vi "Abort Mission and RTH.vi"(8 "Error In":errorcluster, 11 "Aircraft Index":u8) -> (0 "Error Out":errorcluster)   [LabVIEW 2014]
uses:
  Aircraft Information/Sub VI/Get Aircraft Waypoints.vi
  Commands/Mission Planning/MISSION_ITEM SubVI/MISSION_ITEM Jump.vi
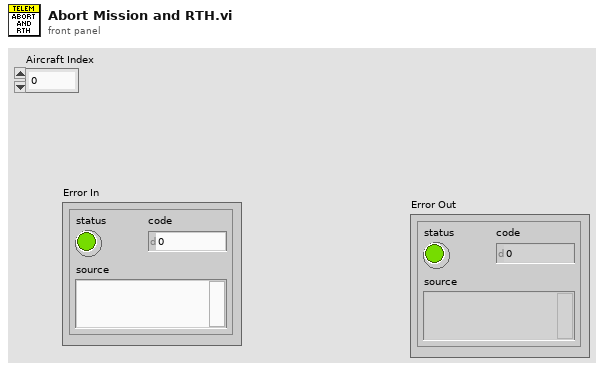
[diagram p1: front panel]
types:
  T1 = typedef "MAVLINK Mav Frame.ctl" = enum8{"GLOBAL", "LOCAL NED", "MISSION", "GLOBAL RELATIVE ALT", "LOCAL ENU", "GLOBAL INT", "GLOBAL RELATIVE ALT INT", "LOCAL OFFSET NED", "BODY NED", "BODY OFFSET NED", "GLOBAL TERRAIN ALT", "GLOBAL TERRAIN ALT INT"}
  T2 = cluster{"target_system":u8, "target_component":u8, "sequence":u16, "frame":T1, "command":u16, "current":bool, "autocontinue":bool, "param1":sgl, "param2":sgl, "param3":sgl, "param4":sgl, "x":sgl, "y":sgl, "z":sgl}[]
  T3 = typedef "MAVLINK Mission Item.ctl" = cluster{"target_system":u8, "target_component":u8, "sequence":u16, "frame":T1, "command":u16, "current":bool, "autocontinue":bool, "param1":sgl, "param2":sgl, "param3":sgl, "param4":sgl, "Lat":sgl, "Lon":sgl, "Altitude (m)":sgl}
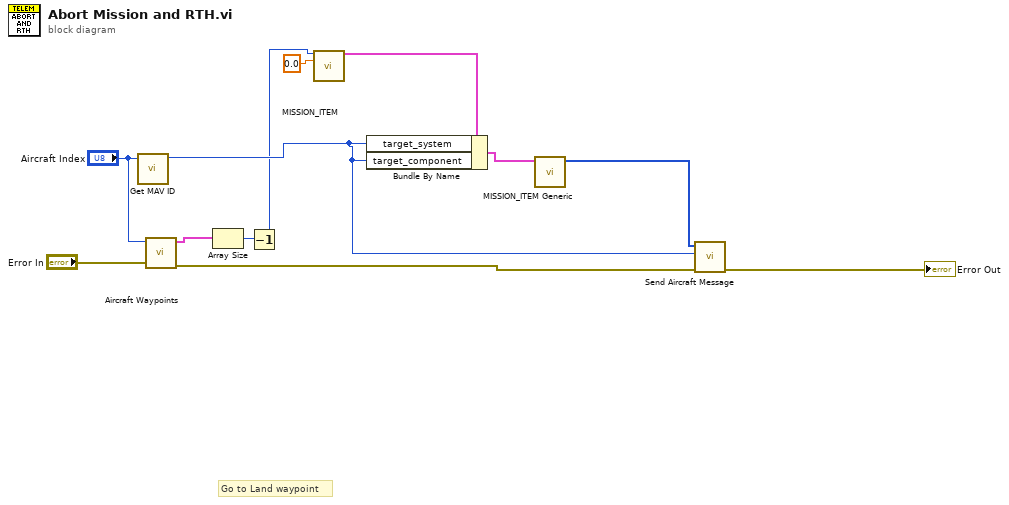
[diagram p0: block diagram]
diagram:
  # "Go to Land waypoint"
  n1 = call "Get MAV ID.vi"("Aircraft Index"="Aircraft Index") -> ("Aircraft ID"=w9:u8)  [unwired: 10 in]
  n2 = call-poly "Aircraft Waypoints.vi"("Error In"="Error In", "Aircraft ID"="Aircraft Index") -> ("Error Out"=w6:errorcluster, "Waypoints Out"=w4:T2)  [unwired: 8 in]
  n3 = Array Size(array=w4) -> (size(s)=w3:i32)
  n4 = Decrement(x=w3) -> (x-1=w2:i32)
  n5 = call-poly "MISSION_ITEM.vi"("Waypoint to jump to"=w2, "Number of times to repeat"=sgl 0.0) -> ("Mission Item"=w12:T3)  [unwired: 13 in]
  n6 = Bundle By Name(cluster=w12, "target_system"=w9, "target_component"=w9) -> (w11:T3)
  n7 = call "MISSION_ITEM Generic.vi"("MISSION_ITEM"=w11) -> ("MAVLink Message"=w10:u8[])  [unwired: 10 in]
  n8 = call "Send Aircraft Message.vi"("error in (no error)"=w6, "Aircraft ID"=w9, "MAVLink Message"=w10) -> ("error out"=→"Error Out":errorcluster)  [unwired: 8 in]
